vi "Write Configuration File.vi"(8 "error in (no error)":errorcluster, 11 "Example Instrument in":refnum<class "Example Instrument.lvclass">) -> (0 "error out":errorcluster, 3 "Example Instrument out":refnum<class "Example Instrument.lvclass">)   [LabVIEW 2016, in "Example Instrument.lvclass"]
uses:
  Example Instrument.lvclass
  C:/user/patrick/hg/levylab_inst del/lvsrc/SMOs/Instrument/Instrument.lvclass
  Instrument/Instrument.lvclass/Instrument.ctl
  Example Instrument.lvclass/Example Instrument.ctl
  Configuration/Configuration.lvclass
  Instrument/Instrument.lvclass
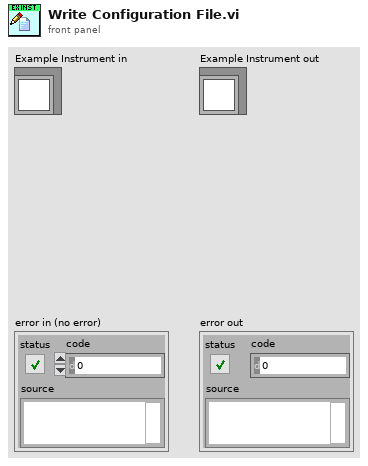
[diagram p1: front panel]
types:
  T1 = typedef "Example Instrument.lvclass/Configuration--Cluster.ctl" = cluster{"Example Setting 1":dbl, "Example Setting 2":dbl, "Example Setting 3":string}
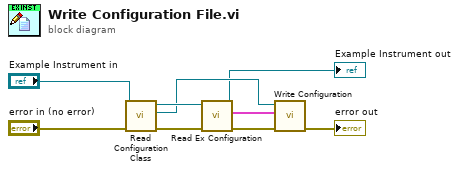
[diagram p0: block diagram]
diagram:
  n1 = call "Read Configuration Class.vi"("error in (no error)"="error in (no error)", "Instrument in"="Example Instrument in") -> ("error out"=w4:errorcluster, "Configuration.lvclass"=w7:refnum<class "Configuration.lvclass">, "Instrument out"=w8:refnum<class "Example Instrument.lvclass">)  [unwired: 7 in]
  n2 = call "Read Ex Configuration.vi"("error in (no error)"=w4, "Example Instrument in"=w8) -> ("error out"=w3:errorcluster, "Ex Configuration"=w9:T1, "Example Instrument out"=→"Example Instrument out":refnum<class "Example Instrument.lvclass">)  [unwired: 7 in]
  n3 = call "Write Configuration.vi"("error in (no error)"=w3, "Variant"=w9, "Configuration in"=w7) -> ("error out"=→"error out":errorcluster)  [unwired: 7 in, 1 out]
